vi "insert.vi"(8 "error in (no error)":errorcluster, 11 "DataCollectionDL110128Streaming in":refnum<class "DataCollectionDL110128Streaming.lvclass">) -> (0 "error out":errorcluster, 3 "DataCollectionDL110128Streaming out":refnum<class "DataCollectionDL110128Streaming.lvclass">)   [LabVIEW 2010, in "DataCollectionDL110128Streaming.lvclass"]
uses:
  DataCollectionDL110128Streaming.lvclass
  DataCollectionDL110128Streaming.lvclass/DataCollectionDL110128Streaming.ctl
  common/classes/GenericComponent/GenericComponent/class_data.vi
  common/classes/GenericComponent/GenericComponent/GenericComponent.lvclass
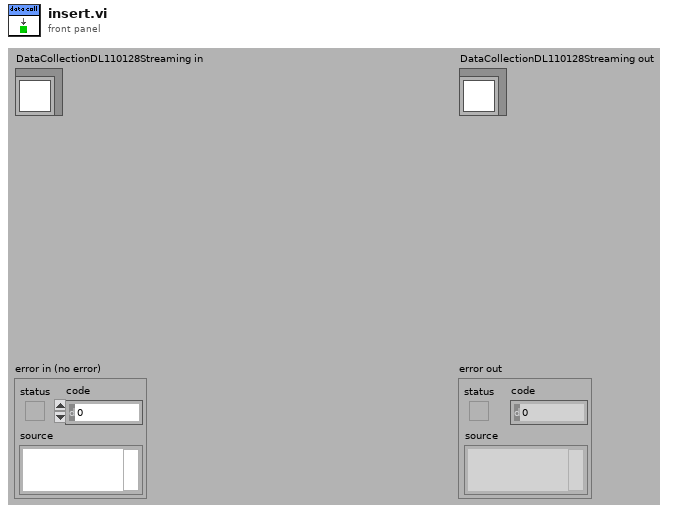
[diagram p1: front panel]
types:
  T1 = enum16{"open", "replace", "create", "open or create", "replace or create", "replace or create with confirmation"}
  T2 = typedef "pixel_raw_data_array.ctl" = dbl[][]
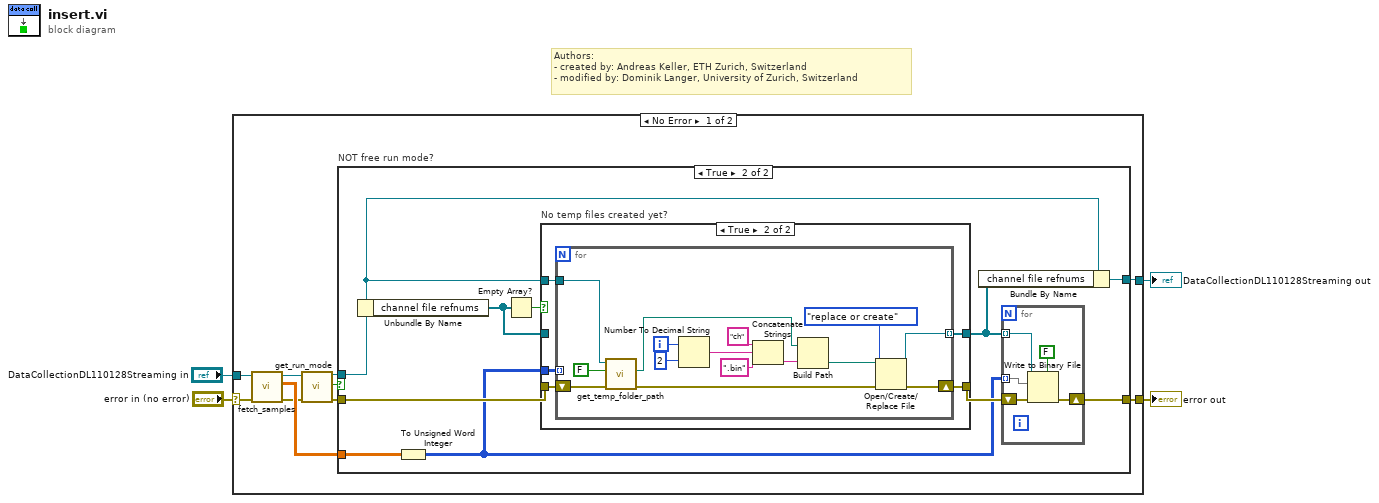
[diagram p0: block diagram]
diagram:
  # "Authors: \n- created by: Andreas Keller, ETH Zurich, Switzerland\n- modified by: Dominik Langer, University of Zurich, Switzerland"
  n1 = case shown="No Error" "error in (no error)" {
    selector: "error in (no error)" -> [w13 w55]
    tunnel: [w12 w55] -> w3
    tunnel: [w11 w54] -> w1
    tunnel: "DataCollectionDL110128Streaming in" -> [w14 w54]
    frame No Error {
      n2 = call-dynamic "fetch_samples.vi"("error in (no error)"=w13, "GenericToplevelComponent in"=w14) -> ("error out"=w9:errorcluster, "channels raw data block"=w10:T2, "GenericToplevelComponent out"=w7:refnum<class "DataCollectionDL110128Streaming.lvclass">)  [unwired: 6 in, 1 out]
      n3 = call "get_run_mode.vi"("error in (no error)"=w9, "GenericPlugin in"=w7) -> ("error out"=w8:errorcluster, "GenericPlugin out"=w5:refnum<class "DataCollectionDL110128Streaming.lvclass">, "is NOT free run?"=w6:bool)  [unwired: 5 in, 2 out]
      n4 = case "NOT free run mode?" shown="True" w6 {
        tunnel: [w16 w24] -> w12
        tunnel: [w15 w22] -> w11
        tunnel: w10 -> [_ w18]
        tunnel: w8 -> [w16 w20]
        tunnel: w5 -> [w15 w19]
        frame False {
        }
        frame True {
          n5 = Unbundle By Name(w19) -> ("channel file refnums"=w26:refnum<file>[])
          n6 = To Unsigned Word Integer(number=w18) -> (unsigned 16bit integer=w17:u16[][])
          n7 = Empty Array?(array=w26) -> (empty?=w21:bool)
          n8 = case "No temp files created yet?" shown="True" w21 {
            tunnel: w20 -> [w33 w38]
            tunnel: [w33 w37] -> w25
            tunnel: w17 -> [_ w36]
            tunnel: w26 -> [w32 _]
            tunnel: [w32 w35] -> w23
            tunnel: w19 -> [_ w34]
            frame False {
            }
            frame True {
              n9 = for {
                shift-right: [w53] -> w37
                shift-left: w38 -> [w52]
                tunnel: w36 -> [_] mode=indexing
                tunnel: [w51] -> w35 mode=indexing
                tunnel: w34 -> [w50]
                i -> [w46]
                n10 = call-dynamic "get_temp_folder_path.vi"("error in (no error)"=w52, "flush?"=FALSE, "GenericComponent in"=w50) -> ("error out"=w40:errorcluster, "temp path"=w39:path)  [unwired: 6 in, 1 out]
                n11 = Number To Decimal String(number=w46, width (-)=i16 2) -> (decimal integer string=w44:string)
                n12 = Concatenate Strings("ch", w44, ".bin") -> (w43:string)
                n13 = Build Path(base path=w39, name or relative path=w43) -> (appended path=w47:path)
                n14 = Open/Create/Replace File(file path (use dialog)=w47, error in=w40, operation (0:open)=T1."replace or create") -> (refnum out=w51:refnum<file>, error out=w53:errorcluster)  [unwired: 3 in, 1 out]
              }
            }
          }
          n15 = Bundle By Name(cluster=w19, "channel file refnums"=w23) -> (w22:refnum<class "DataCollectionDL110128Streaming.lvclass">)
          n16 = for {
            tunnel: w23 -> [w29] mode=indexing
            tunnel: w17 -> [w27] mode=indexing
            shift-right: [w30] -> w24
            shift-left: w25 -> [w31]
            n17 = Write to Binary File(file (use dialog)=w29, data=w27, error in=w31, 5:FALSE ("prepend array or string size? (T)")) -> (error out=w30:errorcluster)  [unwired: 2 in, 2 out]
          }
        }
      }
    }
    frame Error {
    }
  }
  "error out" <- w3
  "DataCollectionDL110128Streaming out" <- w1
